vi "Teleop.vi"(10 "Match Info":T1={"Autonomous Elapsed Seconds"=0.0, "TeleOp Elapsed Seconds"=0.0, "Disabled Elapsed Seconds"=0.0, "Visited Autonomous"=FALSE, "Visited TeleOp"=FALSE, "Visited Disabled"=FALSE, "Autonomous Settings"={"Autonomous Style"=enum."Independent", "VI Refnum"=refnum}}, 11 "Call Context":T2) -> ()   [LabVIEW 2014]
doc: "This VI is called for each TeleOp packet received from the DS where the robot is not disabled. It is often used to read from the joysticks and update I/O or to update setpoints for timed control loops. It should complete and return within 20 milliseconds or it may miss DS packets."
uses:
  <vilib>/Rock Robotics/WPI/DriverStation/WPI_DriverStationDerivedRobotMode.ctl
  <vilib>/Rock Robotics/WPI/DriverStation/WPI_DriverStationMatch Info.ctl
  Utilities/Refname.ctl
  Input/JoyCurve Axes.ctl
  Utilities/RefnameToString.vi
  <vilib>/Rock Robotics/WPI/Joystick/WPI_JoystickGetSetRefNum.vi
  Robot Global Data.vi
  <vilib>/Rock Robotics/Network Tables/SD Read Number.vi
panel:
  # "Operator Controller"
  # "Driver Controller"
  # "Controller"
  # "Controller"
  # "Half-Drive"
  # "Clapper Out"
  # "Motor Ramp"
  # "Clapper In"
  # "Elevator \nSafety\nOverride"
  # "Elevator Bin Modifier"
  # "Lower Arms"
  # "Raise Arms"
  # "Manual Raise Arms"
  # "Feeder pickup"
  # "Elevator Up"
  # "Manual Clapper Out"
  # "Manual Clapper In"
  # "Wiper"
  # "Feeder up"
  # "Manual Lower Arms"
  # "Elevator Pickup"
  # "Feeder down"
  # "Elevator Down"
  # "Elevator Reset"
  # "Strafe"
  # "Rotating"
  # "Fwd/Back"
  # "Elevator"
  # "Arm rollers (in / out)"
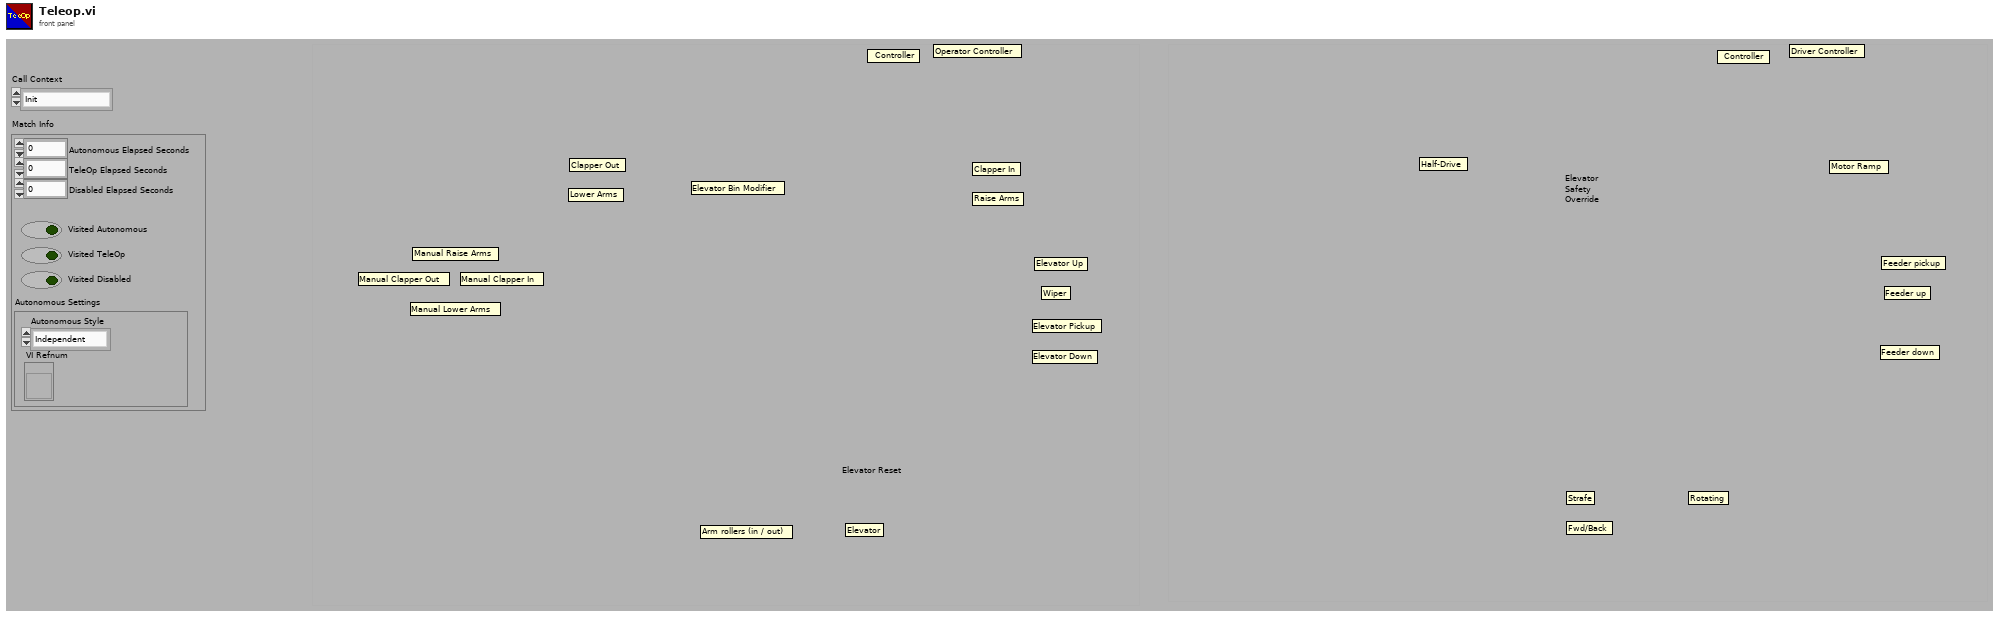
[diagram p1: front panel]
types:
  T1 = typedef "WPI_DriverStationMatch Info.ctl" = cluster{"Autonomous Elapsed Seconds":dbl, "TeleOp Elapsed Seconds":dbl, "Disabled Elapsed Seconds":dbl, "Visited Autonomous":bool, "Visited TeleOp":bool, "Visited Disabled":bool, "Autonomous Settings":cluster{"Autonomous Style":enum16{"Iterative", "Independent"}, "VI Refnum":refnum<vi>}}
  T2 = typedef "WPI_DriverStationDerivedRobotMode.ctl" = enum16{"Init", "Execute", "Stop"}
  T3 = typedef "JoyCurve Axes.ctl" = cluster{"Left Joystick X":dbl, "Left Joystick Y":dbl, "Right Joystick X":dbl, "Right Joystick Y":dbl}
  T4 = typedef "Refname.ctl" = enum16{"Gamepad 1", "Gamepad 2", "Drive Motors", "Strafe Motor", "Arm Clapper Motor", "Arm Angle", "Arm Belt Left", "Arm Belt Right", "Elevator 1", "Elevator 2", "Wiper"}
  T5 = typedef "WPI_JoystickDevRef.ctl" = cluster{"Device":T6}
  T6 = typedef "WPI_JoystickDeviceEnum.ctl" = enum16{"USB 0", "USB 1", "USB 2", "USB 3", "USB 4", "USB 5"}
  T7 = cluster{"upper limit":dbl, "upper limit":dbl, "upper limit":dbl, "upper limit":dbl}
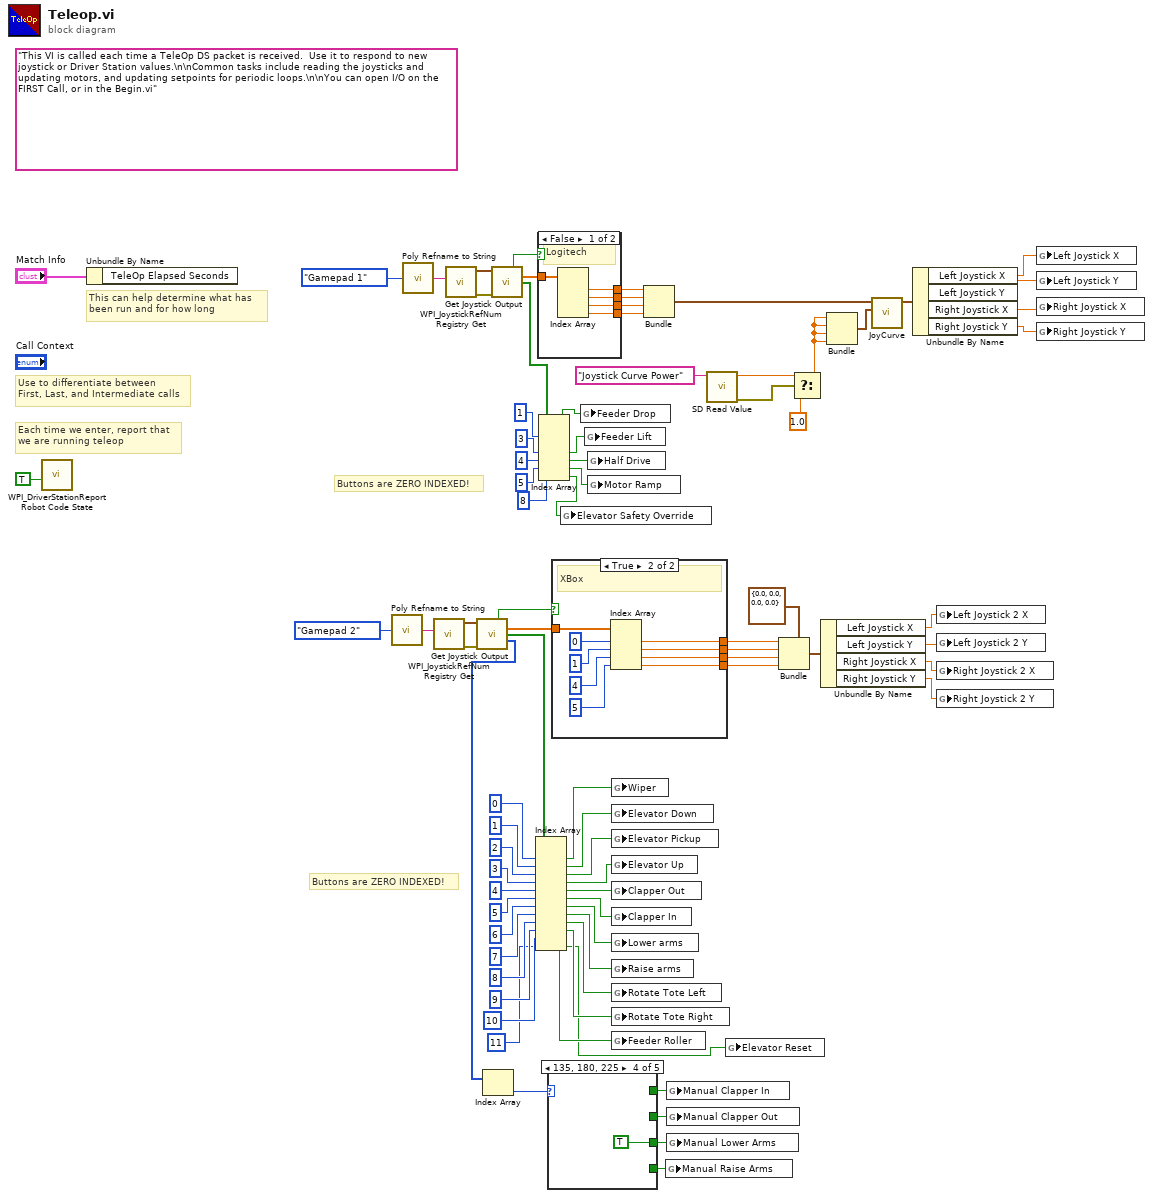
[diagram p0: block diagram]
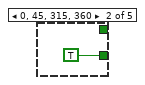
[diagram p3: hidden frame]
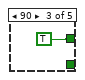
[diagram p4: hidden frame]
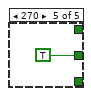
[diagram p5: hidden frame]
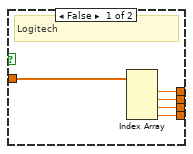
[diagram p6: hidden frame]
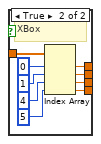
[diagram p7: hidden frame]
diagram:
  (unwired) "This VI is called each time a TeleOp DS packet is received.  Use it to respond to new joystick or Driver Station values.\n\nCommon tasks include reading the joysticks and updating motors, and updating setpoints for periodic loops.\n\nYou can open I/O on the FIRST Call, or in the Begin.vi"
  # "Buttons are ZERO INDEXED!"
  # "Buttons are ZERO INDEXED!"
  # "Each time we enter, report that\nwe are running teleop"
  # "Use to differentiate between\nFirst, Last, and Intermediate calls"
  # "This can help determine what has\nbeen run and for how long"
  n1 = call <vilib>:"WPI_DriverStationReport Robot Code State.vi"("TeleOp"=TRUE ("Autonomous")) -> ()  [unwired: 10 in, 1 out]
  n2 = Unbundle By Name("Match Info") -> ()  [unwired: 1 out]
  n3 = call-poly "Poly Refname to String.vi"("Enum"=Refname."Gamepad 2") -> ("Refname"=w78:string)
  n4 = call-poly "Poly Refname to String.vi"("Enum"=Refname."Gamepad 1" ("Refname")) -> ("Refname"=w80:string)
  n5 = call <vilib>:"WPI_JoystickRefNum Registry Get.vi"("refnum name"=w78) -> ("error out"=w72:errorcluster, "JoystickDevRef"=w76:T5)  [unwired: 9 in]
  n6 = call <vilib>:"WPI_JoystickRefNum Registry Get.vi"("refnum name"=w80) -> ("error out"=w73:errorcluster, "JoystickDevRef"=w77:T5)  [unwired: 9 in]
  n7 = call "Get Joystick Output.vi"("JoystickDevRef"=w76, "error in (no error)"=w72) -> ("XBox?"=w55:bool, "Axes"=w54:dbl[], "Buttons"=w61:bool[], "POVs"=w27:i16[])  [unwired: 8 in, 2 out]
  n8 = Index Array(array=w27) -> (element=w26:i16)  [unwired: 1 in]
  n9 = call "Get Joystick Output.vi"("JoystickDevRef"=w77, "error in (no error)"=w73) -> ("XBox?"=w74:bool, "Axes"=w75:dbl[], "Buttons"=w47:bool[])  [unwired: 8 in, 3 out]
  n10 = Index Array(array=w61, index #1=0 ("index"), index #2=1 ("index"), index #3=2 ("index"), index #4=3 ("index"), index #5=4 ("index"), index #6=5 ("index"), index #7=6 ("index"), index #8=7 ("index"), index #9=8 ("index"), index #10=9 ("index"), index #11=10 ("index"), index #12=11 ("index")) -> (element #1=w5:bool, element #2=w32:bool, element #3=w30:bool, element #4=w31:bool, element #5=w17:bool, element #6=w16:bool, element #7=w29:bool, element #8=w28:bool, element #9=w19:bool, element #10=w18:bool, element #11=w8:bool, element #12=w3:bool)
  n11 = case shown="False" w74 {
    tunnel: w75 -> [w87 w96]
    tunnel: [w86 w92] -> w70
    tunnel: [w85 w90] -> w68
    tunnel: [w84 w91] -> w69
    tunnel: [w83 w93] -> w71
    frame False {
      # "Logitech"
      n12 = Index Array(array=w87) -> (element #1=w83:dbl, element #2=w86:dbl, element #3=w84:dbl, element #4=w85:dbl)  [unwired: 4 in]
    }
    frame True {
      # "XBox"
      n13 = Index Array(array=w96, index #1=0 ("index"), index #2=1 ("index"), index #3=4 ("index"), index #4=5 ("index")) -> (element #1=w93:dbl, element #2=w92:dbl, element #3=w91:dbl, element #4=w90:dbl)
    }
  }
  n14 = Index Array(array=w47, index #1=1 ("index"), index #3=3 ("index"), index #4=4 ("index"), index #5=5 ("index"), index #6=8 ("index")) -> (element #1=w6:bool, element #3=w10:bool, element #4=w11:bool, element #5=w12:bool, element #6=w1:bool)  [unwired: 1 in, 1 out]
  n15 = case shown="135, 180, 225" w26 {
    tunnel: [_ _ TRUE _ _] -> w25
    tunnel: [_ _ _ _ TRUE] -> w24
    tunnel: [_ _ _ TRUE _] -> w23
    tunnel: [_ TRUE _ _ _] -> w22
    frame -1, Default {
    }
    frame 0, 45, 315, 360 {
    }
    frame 90 {
    }
    frame 135, 180, 225 {
    }
    frame 270 {
    }
  }
  n16 = case shown="True" w55 {
    tunnel: w54 -> [w101 w114]
    tunnel: [w104 w112] -> w57
    tunnel: [w102 w110] -> w56
    tunnel: [w103 w111] -> w58
    tunnel: [w105 w113] -> w59
    frame False {
      # "Logitech"
      n17 = Index Array(array=w101) -> (element #1=w105:dbl, element #2=w104:dbl, element #3=w103:dbl, element #4=w102:dbl)  [unwired: 4 in]
    }
    frame True {
      # "XBox"
      n18 = Index Array(array=w114, index #1=0 ("index"), index #2=1 ("index"), index #3=4 ("index"), index #4=5 ("index")) -> (element #1=w113:dbl, element #2=w112:dbl, element #3=w111:dbl, element #4=w110:dbl)
    }
  }
  n19 = global write "Robot Global Data.vi" "Elevator Safety Override"(w1) -> ()
  n20 = global write "Robot Global Data.vi" "Feeder Drop"(w6) -> ()
  n21 = global write "Robot Global Data.vi" "Feeder Lift"(w10) -> ()
  n22 = global write "Robot Global Data.vi" "Half Drive"(w11) -> ()
  n23 = global write "Robot Global Data.vi" "Motor Ramp"(w12) -> ()
  n24 = global write "Robot Global Data.vi" "Wiper"(w5) -> ()
  n25 = global write "Robot Global Data.vi" "Elevator Down"(w32) -> ()
  n26 = global write "Robot Global Data.vi" "Elevator Pickup"(w30) -> ()
  n27 = global write "Robot Global Data.vi" "Elevator Up"(w31) -> ()
  n28 = global write "Robot Global Data.vi" "Clapper Out"(w17) -> ()
  n29 = global write "Robot Global Data.vi" "Clapper In"(w16) -> ()
  n30 = global write "Robot Global Data.vi" "Lower arms"(w29) -> ()
  n31 = global write "Robot Global Data.vi" "Raise arms"(w28) -> ()
  n32 = global write "Robot Global Data.vi" "Rotate Tote Left"(w19) -> ()
  n33 = global write "Robot Global Data.vi" "Rotate Tote Right"(w18) -> ()
  n34 = global write "Robot Global Data.vi" "Feeder Roller"(w8) -> ()
  n35 = Bundle("upper limit"=w71, "upper limit"=w70, "upper limit"=w69, "upper limit"=w68) -> (w67:T7)  [unwired: 1 in]
  n36 = global write "Robot Global Data.vi" "Manual Raise Arms"(w22) -> ()
  n37 = global write "Robot Global Data.vi" "Manual Clapper In"(w25) -> ()
  n38 = global write "Robot Global Data.vi" "Manual Clapper Out"(w24) -> ()
  n39 = global write "Robot Global Data.vi" "Manual Lower Arms"(w23) -> ()
  n40 = call-poly <vilib>:"SD Read Value.vi"("Name"="Joystick Curve Power") -> ("error out"=w36:errorcluster, "Numeric"=w35:dbl)  [unwired: 8 in, 1 out]
  n41 = global write "Robot Global Data.vi" "Elevator Reset"(w3) -> ()
  n42 = Bundle(cluster=T3 {"Left Joystick X"=0.0, "Left Joystick Y"=0.0, "Right Joystick X"=0.0, "Right Joystick Y"=0.0} ("Axes"), "Left Joystick X"=w59, "Left Joystick Y"=w57, "Right Joystick X"=w58, "Right Joystick Y"=w56) -> (w53:T3)
  n43 = Select(t=w35, s=w36, f=1.0 ("t")) -> (s? t:f=w34:dbl)
  n44 = Unbundle By Name(w53) -> ("Left Joystick X"=w51:dbl, "Left Joystick Y"=w50:dbl, "Right Joystick X"=w49:dbl, "Right Joystick Y"=w48:dbl)
  n45 = Bundle("t"=w34, "t"=w34, "t"=w34, "t"=w34) -> (w45:cluster{"t":dbl, "t":dbl, "t":dbl, "t":dbl})  [unwired: 1 in]
  n46 = call "JoyCurve.vi"("Powers"=w45, "Axes"=w67) -> ("Axes Out"=w66:T3)  [unwired: 8 in, 1 out]
  n47 = Unbundle By Name(w66) -> ("Left Joystick X"=w65:dbl, "Left Joystick Y"=w64:dbl, "Right Joystick X"=w63:dbl, "Right Joystick Y"=w62:dbl)
  n48 = global write "Robot Global Data.vi" "Left Joystick 2 X"(w51) -> ()
  n49 = global write "Robot Global Data.vi" "Left Joystick 2 Y"(w50) -> ()
  n50 = global write "Robot Global Data.vi" "Right Joystick 2 X"(w49) -> ()
  n51 = global write "Robot Global Data.vi" "Right Joystick 2 Y"(w48) -> ()
  n52 = global write "Robot Global Data.vi" "Left Joystick X"(w65) -> ()
  n53 = global write "Robot Global Data.vi" "Left Joystick Y"(w64) -> ()
  n54 = global write "Robot Global Data.vi" "Right Joystick X"(w63) -> ()
  n55 = global write "Robot Global Data.vi" "Right Joystick Y"(w62) -> ()
